vi "_Split Response After Out Of Tolerance Reliability.vi"(0 "Input String":string) -> (1 "Reliability out":i32, 2 "Out Of Tolerance":i32, 3 "Response out":string[](array[string]))   [LabVIEW 2015, in "Rohde&Schwarz CMP LR WPAN Measurement.lvlib"]
uses:
  <instrlib>/Rohde&Schwarz CMP LR WPAN Measurement/Rohde&Schwarz CMP LR WPAN Measurement.lvlib
  <instrlib>/Rohde&Schwarz CMP LR WPAN Measurement/Private/rsidr_core.llb/rsidr_core.lvlib
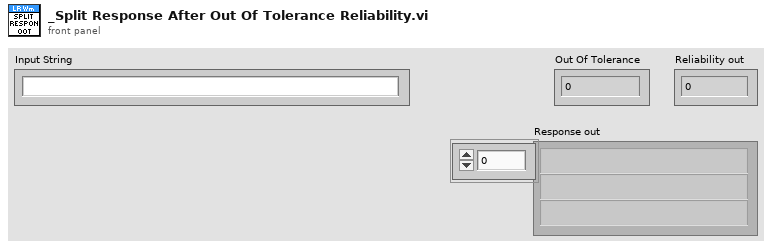
[diagram p1: front panel]
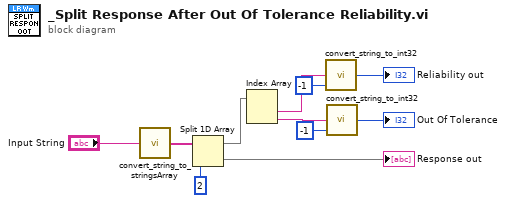
[diagram p0: block diagram]
diagram:
  n1 = call <instrlib>:"convert_string_to_stringsArray.vi"("String in"="Input String") -> ("string array out"=w8:string[])  [unwired: 3 in, 1 out]
  n2 = Split 1D Array(array=w8, index=2) -> (first subarray=w1:string[], second subarray=→"Response out":string[])
  n3 = Index Array(array=w1) -> (element #1=w7:string, element #2=w4:string)  [unwired: 2 in]
  n4 = call <instrlib>:"convert_string_to_int32.vi"("default (0)"=-1 ("default (0 I32)"), "String in"=w7) -> ("int32 value out"=→"Reliability out":i32)  [unwired: 3 in]
  n5 = call <instrlib>:"convert_string_to_int32.vi"("default (0)"=-1 ("default (0 I32)"), "String in"=w4) -> ("int32 value out"=→"Out Of Tolerance":i32)  [unwired: 3 in]
